vi "Agilent34420-V y HP34401A-R.vi"() -> ()   [LabVIEW 2014]
uses:
  <vilib>/Utility/file.llb/Write To Spreadsheet File (string).vi
  Gonzalo/INTI/Gonzalo/agilent34420_medicion_de_cosa_turbia/Program Files/National Instruments/LabVIEW 2014/instr.lib/Agilent 34401/Agilent 34401.lvlib
panel:
  in  "NPLC Res":sgl(ring)=2.0 format="%_1f" items=["200", "100", "20", "10", "2", "1", ".2", "0.02"]
  out "Res":dbl[](graph)
  in  "GPIB mult 2":refnum<visa-resource-name>="GPIB0::14::INSTR"
  in  "error 2":errorcluster
  in  "t esp medic Res":dbl
  in  "RESOL Res":dbl
  in  "RANGE Res (O)":dbl=0.1
  out "medic Res":dbl[](array[numeric]) format="%#.10e"
  out "Medicion Res":string[](array[string])
  out "Medicion CH1":string[](array[string])
  out "Tmed":string[](array[string])
  out "new file path (Not A Path if cancelled)":path
  out "tiempo transcurrido (s)":dbl
  out "tiempo inicio":timestamp format="%<%H:%M:%S%1u>T"
  in  "t esp medic CH1":dbl
  in  "NPLC CH1":sgl(ring)=2.0 format="%_1f" items=["200", "100", "20", "10", "2", "1", ".2", "0.02"]
  in  "RESOL CH1":dbl
  in  "RANGE CH1 (V)":dbl=0.1
  in  "file path (dialog if empty)":path=path "C:/Users/INTI/Desktop/Gonzalo/INTI/Gonzalo/agilent34420_medicion_de_cosa_turbia/mediciones"
  out "Volt":dbl[](graph)
  out "medic ch 1":dbl[](array[numeric]) format="%#.10e"
  in  "termina medic":bool
  out "Boolean":bool
  in  "empieza medic":bool
  in  "error":errorcluster
  in  "GPIB mult":refnum<visa-resource-name>="GPIB0::13::INSTR"
  # "Notas: el programa mide en forma alternada el canal 1 y 2 del multímetro con los rangos y NPLC seleccionados.\n1- seleccionar GPIB addrs\n2- selccionar RANGE y NPLC de los canales, puede elegirse un file path o dejarlo en blanco (al final se pedirá archivo de datos a grabar).\n3- click en MEDIR para comenzar la medición\n4- click en TERMINAR para finalizarla, se solicita file path en este punto de no haberlo seleccionado previamente."
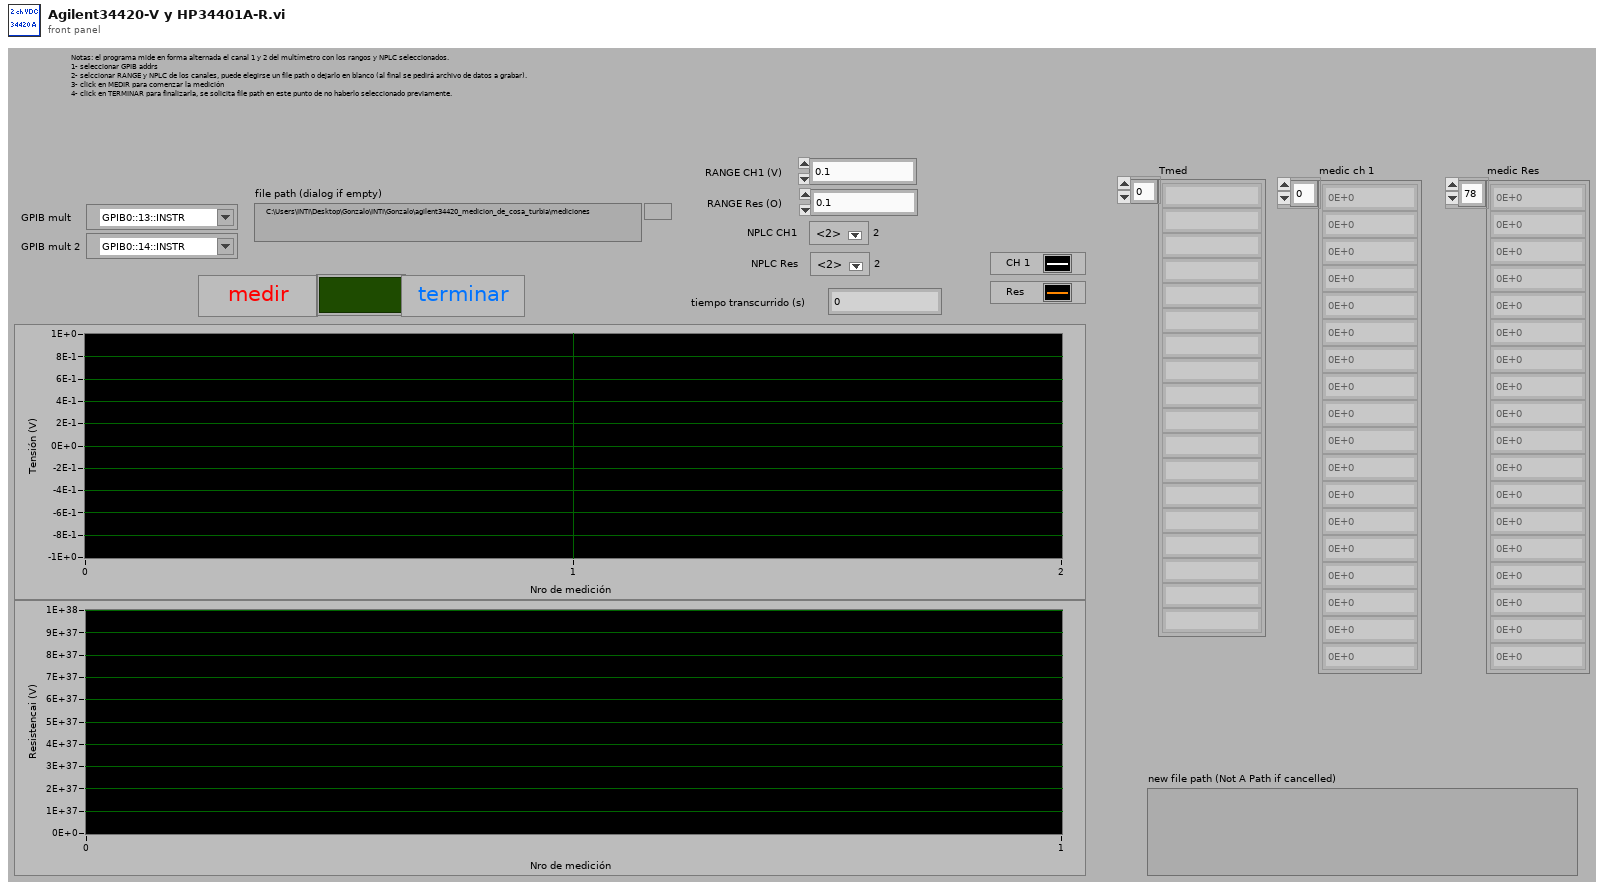
[diagram p1: front panel]
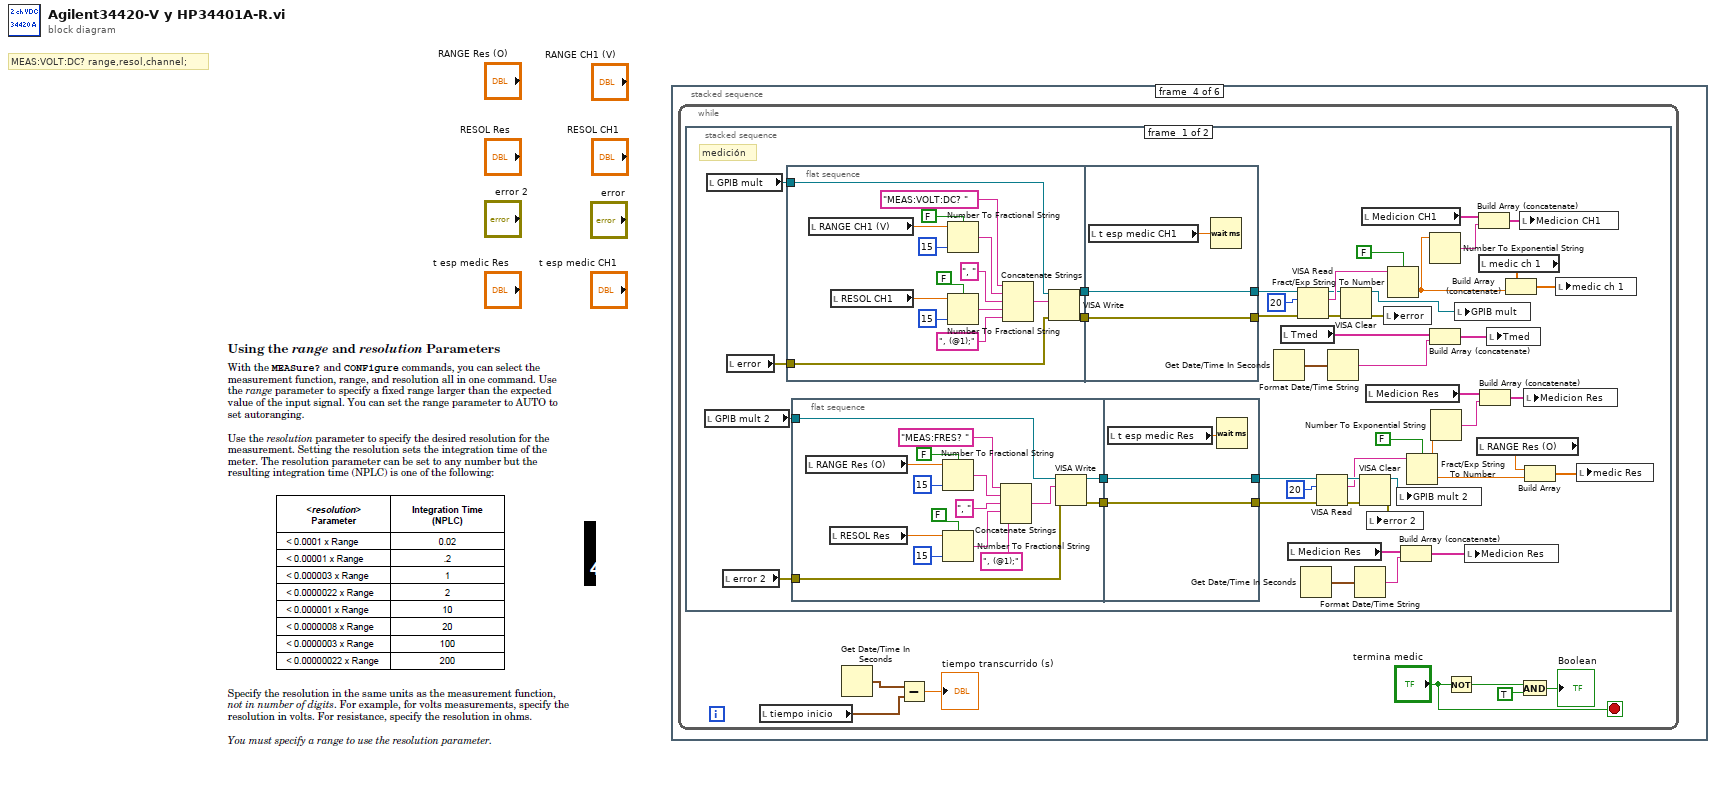
[diagram p0: block diagram]
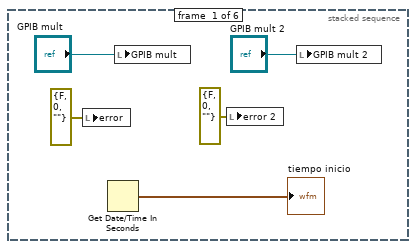
[diagram p2: hidden frame]
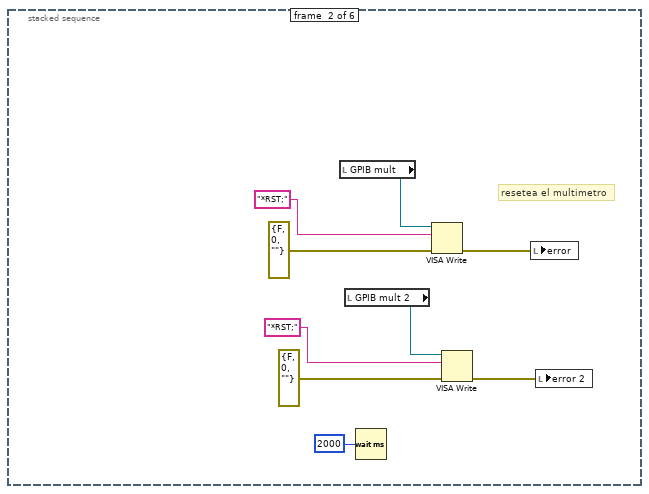
[diagram p3: hidden frame]
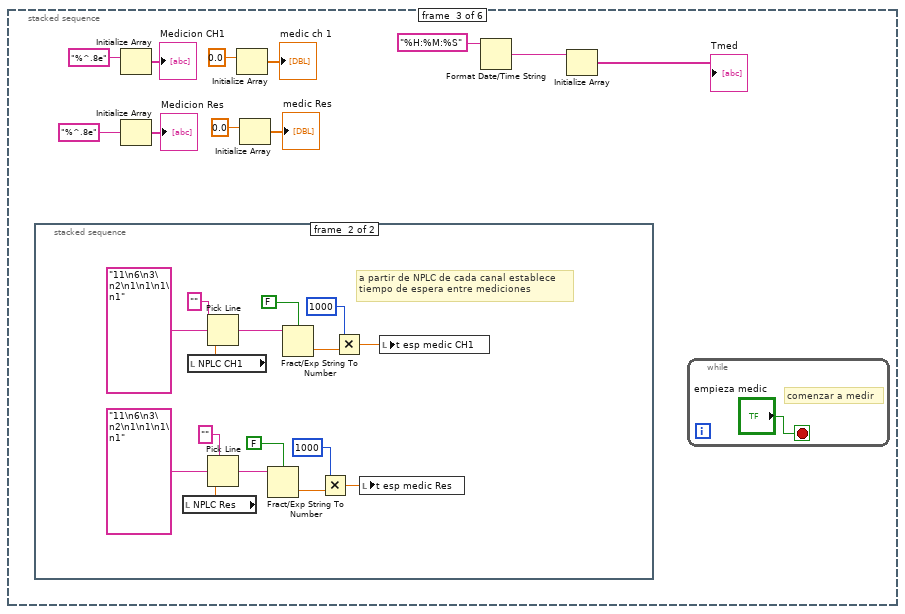
[diagram p4: hidden frame]
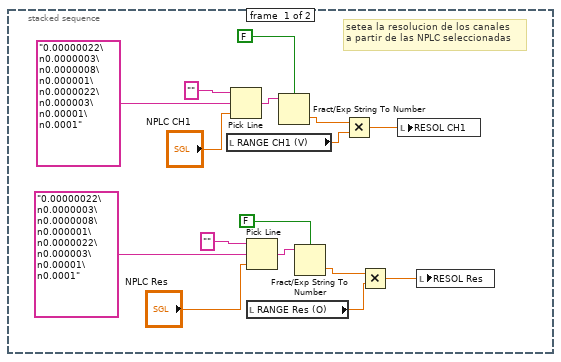
[diagram p5: hidden frame]
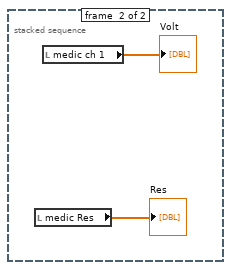
[diagram p6: hidden frame]
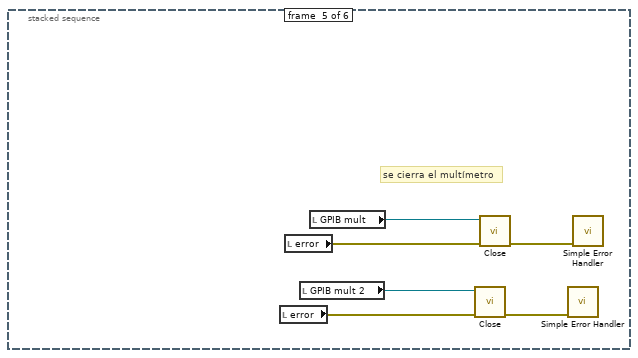
[diagram p7: hidden frame]
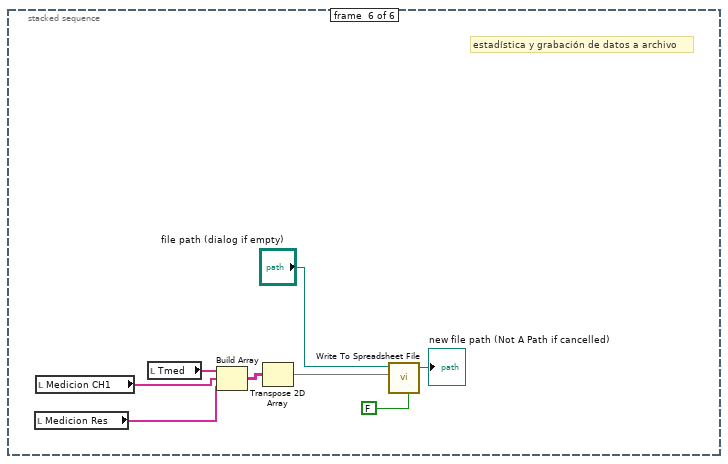
[diagram p8: hidden frame]
diagram:
  # "MEAS:VOLT:DC? range,resol,channel;"
  n1 = stacked-sequence {
    frame #0 {
      n2 = local write "error"(errorcluster {"status"=FALSE, "code"=0, "source"=""} ("error in (no error)")) -> ()
      n3 = Get Date/Time In Seconds() -> (seconds since 1Jan1904=→"tiempo inicio":timestamp)
      n4 = local write "GPIB mult"("GPIB mult") -> ()
      n5 = local write "error 2"(errorcluster {"status"=FALSE, "code"=0, "source"=""} ("error in (no error)")) -> ()
      n6 = local write "GPIB mult 2"("GPIB mult 2") -> ()
    }
    frame #1 {
      # "resetea el multimetro"
      n7 = local read "GPIB mult"() -> (w14:refnum<visa-resource-name>)
      n8 = local read "GPIB mult 2"() -> (w6:refnum<visa-resource-name>)
      n9 = Wait (ms)(milliseconds to wait=u32 2000) -> ()  [unwired: 1 out]
      n10 = VISA Write(VISA resource name=w14, write buffer="*RST;", error in (no error)=errorcluster {"status"=FALSE, "code"=0, "source"=""}) -> (error out=w11:errorcluster)  [unwired: 2 out]
      n11 = VISA Write(VISA resource name=w6, write buffer="*RST;", error in (no error)=errorcluster {"status"=FALSE, "code"=0, "source"=""}) -> (error out=w9:errorcluster)  [unwired: 2 out]
      n12 = local write "error"(w11) -> ()
      n13 = local write "error 2"(w9) -> ()
    }
    frame #2 {
      n14 = stacked-sequence {
        frame #0 {
          # "setea la resolucion de los canales \na partir de las NPLC seleccionadas"
          n15 = local read "RANGE CH1 (V)"() -> (w41:dbl)
          n16 = Pick Line(string ("")="", multi-line string="0.00000022\n0.0000003\n0.0000008\n0.000001\n0.0000022\n0.000003\n0.00001\n0.0001", line index="NPLC CH1") -> (output string=w37:string)
          n17 = Pick Line(string ("")="", multi-line string="0.00000022\n0.0000003\n0.0000008\n0.000001\n0.0000022\n0.000003\n0.00001\n0.0001", line index="NPLC Res") -> (output string=w32:string)
          n18 = local read "RANGE Res (O)"() -> (w27:dbl)
          n19 = Fract/Exp String To Number(use system decimal point (T)=FALSE, string=w37) -> (number=w36:dbl)  [unwired: 2 in, 1 out]
          n20 = Fract/Exp String To Number(use system decimal point (T)=FALSE, string=w32) -> (number=w33:dbl)  [unwired: 2 in, 1 out]
          n21 = Multiply(x=w36, y=w41) -> (x*y=w40:dbl)
          n22 = Multiply(x=w33, y=w27) -> (x*y=w28:dbl)
          n23 = local write "RESOL CH1"(w40) -> ()
          n24 = local write "RESOL Res"(w28) -> ()
        }
        frame #1 {
          # "a partir de NPLC de cada canal establece\ntiempo de espera entre mediciones"
          n25 = local read "NPLC Res"() -> (w42:sgl)
          n26 = local read "NPLC CH1"() -> (w50:sgl)
          n27 = Pick Line(string ("")="", multi-line string="11\n6\n3\n2\n1\n1\n1\n1", line index=w50) -> (output string=w57:string)
          n28 = Pick Line(string ("")="", multi-line string="11\n6\n3\n2\n1\n1\n1\n1", line index=w42) -> (output string=w49:string)
          n29 = Fract/Exp String To Number(use system decimal point (T)=FALSE, string=w49) -> (number=w46:dbl)  [unwired: 2 in, 1 out]
          n30 = Fract/Exp String To Number(use system decimal point (T)=FALSE, string=w57) -> (number=w54:dbl)  [unwired: 2 in, 1 out]
          n31 = Multiply(x=1000, y=w46) -> (x*y=w44:dbl)
          n32 = Multiply(x=1000, y=w54) -> (x*y=w52:dbl)
          n33 = local write "t esp medic Res"(w44) -> ()
          n34 = local write "t esp medic CH1"(w52) -> ()
        }
      }
      n35 = Initialize Array("%^.8e" ("format (%.3f)")) -> (→"Medicion CH1":string[])  [unwired: 1 in]
      n36 = Initialize Array("%^.8e" ("format (%.3f)")) -> (→"Medicion Res":string[])  [unwired: 1 in]
      n37 = Initialize Array(0.0 ("element")) -> (→"medic ch 1":dbl[])  [unwired: 1 in]
      n38 = Initialize Array(0.0 ("element")) -> (→"medic Res":dbl[])  [unwired: 1 in]
      n39 = Format Date/Time String(time format string (%c)="%H:%M:%S") -> (date/time string=w23:string)  [unwired: 2 in]
      n40 = Initialize Array(w23) -> (→"Tmed":string[])  [unwired: 1 in]
      n41 = while {
        stop <- "empieza medic" stop-if-true
        # "comenzar a medir"
      }
    }
    frame #3 {
      n42 = while {
        stop <- "termina medic" stop-if-true
        n43 = stacked-sequence {
          frame #0 {
            # "medición"
            n44 = local read "GPIB mult 2"() -> (w88:refnum<visa-resource-name>)
            n45 = local read "GPIB mult"() -> (w102:refnum<visa-resource-name>)
            n46 = local read "error 2"() -> (w66:errorcluster)
            n47 = local read "error"() -> (w103:errorcluster)
            n48 = flat-sequence {
              tunnel: w103 -> [w146]
              tunnel: w102 -> [w145]
              tunnel: [w144] -> w99
              tunnel: [w143] -> w98
              tunnel: [w148] -> w100
              tunnel: [w149] -> w101
              tunnel: w99 -> [w149]
              tunnel: w98 -> [w148]
              frame #0 {
                n49 = local read "RANGE CH1 (V)"() -> (w141:dbl)
                n50 = local read "RESOL CH1"() -> (w136:dbl)
                n51 = Number To Fractional String(use system decimal point (T)=FALSE, number=w141, precision (6)=i16 15) -> (F-format string=w139:string)  [unwired: 1 in]
                n52 = Number To Fractional String(use system decimal point (T)=FALSE, number=w136, precision (6)=i16 15) -> (F-format string=w135:string)  [unwired: 1 in]
                n53 = Concatenate Strings("MEAS:VOLT:DC? " ("write buffer"), w139, ", " ("string"), w135, ", (@1);" ("string")) -> (w133:string)
                n54 = VISA Write(VISA resource name=w145, write buffer=w133, error in (no error)=w146) -> (VISA resource name out=w144:refnum<visa-resource-name>, error out=w143:errorcluster)  [unwired: 1 out]
              }
              frame #1 {
                n55 = local read "t esp medic CH1"() -> (w147:dbl)
                n56 = Wait (ms)(milliseconds to wait=w147) -> ()  [unwired: 1 out]
              }
            }
            n57 = flat-sequence {
              tunnel: w88 -> [w116]
              tunnel: [w114] -> w87
              tunnel: [w113] -> w86
              tunnel: w66 -> [w112]
              tunnel: w87 -> [w130]
              tunnel: [w130] -> w69
              tunnel: w86 -> [w129]
              tunnel: [w129] -> w68
              frame #0 {
                n58 = local read "RANGE Res (O)"() -> (w119:dbl)
                n59 = local read "RESOL Res"() -> (w124:dbl)
                n60 = Number To Fractional String(use system decimal point (T)=FALSE, number=w119, precision (6)=i16 15) -> (F-format string=w121:string)  [unwired: 1 in]
                n61 = Number To Fractional String(use system decimal point (T)=FALSE, number=w124, precision (6)=i16 15) -> (F-format string=w125:string)  [unwired: 1 in]
                n62 = Concatenate Strings("MEAS:FRES? " ("write buffer"), w121, ", " ("string"), w125, ", (@1);" ("string")) -> (w115:string)
                n63 = VISA Write(VISA resource name=w116, write buffer=w115, error in (no error)=w112) -> (VISA resource name out=w113:refnum<visa-resource-name>, error out=w114:errorcluster)  [unwired: 1 out]
              }
              frame #1 {
                n64 = local read "t esp medic Res"() -> (w128:dbl)
                n65 = Wait (ms)(milliseconds to wait=w128) -> ()  [unwired: 1 out]
              }
            }
            n66 = Get Date/Time In Seconds() -> (seconds since 1Jan1904=w93:timestamp)
            n67 = local read "Tmed"() -> (w95:string[])
            n68 = local read "Medicion Res"() -> (w79:string[])
            n69 = VISA Read(VISA resource name=w101, byte count=u32 20, error in (no error)=w100) -> (VISA resource name out=w109:refnum<visa-resource-name>, read buffer=w111:string, error out=w108:errorcluster)  [unwired: 1 out]
            n70 = Get Date/Time In Seconds() -> (seconds since 1Jan1904=w81:timestamp)
            n71 = VISA Read(VISA resource name=w68, byte count=u32 20, error in (no error)=w69) -> (VISA resource name out=w71:refnum<visa-resource-name>, read buffer=w70:string, error out=w72:errorcluster)  [unwired: 1 out]
            n72 = Format Date/Time String(seconds (now)=w93) -> (date/time string=w94:string)  [unwired: 2 in]
            n73 = VISA Clear(VISA resource name=w109, error in (no error)=w108) -> (VISA resource name out=w106:refnum<visa-resource-name>, error out=w107:errorcluster)
            n74 = Format Date/Time String(seconds (now)=w81) -> (date/time string=w80:string)  [unwired: 2 in]
            n75 = VISA Clear(VISA resource name=w71, error in (no error)=w72) -> (VISA resource name out=w74:refnum<visa-resource-name>, error out=w73:errorcluster)
            n76 = local read "Medicion CH1"() -> (w91:string[])
            n77 = local read "Medicion Res"() -> (w83:string[])
            n78 = local write "error 2"(w73) -> ()
            n79 = local write "error"(w107) -> ()
            n80 = Fract/Exp String To Number(use system decimal point (T)=FALSE, string=w111) -> (number=w92:dbl)  [unwired: 2 in, 1 out]
            n81 = local write "GPIB mult 2"(w74) -> ()
            n82 = Build Array (concatenate)(w79, w80) -> (w78:string[])
            n83 = Fract/Exp String To Number(use system decimal point (T)=FALSE, string=w70) -> (number=w82:dbl)  [unwired: 2 in, 1 out]
            n84 = Number To Exponential String(number=w92) -> (E-format string=w90:string)  [unwired: 3 in]
            n85 = Build Array (concatenate)(w95, w94) -> (w96:string[])
            n86 = Number To Exponential String(number=w82) -> (E-format string=w84:string)  [unwired: 3 in]
            n87 = local write "GPIB mult"(w106) -> ()
            n88 = local write "Medicion Res"(w78) -> ()
            n89 = local read "RANGE Res (O)"() -> (w67:dbl)
            n90 = Build Array (concatenate)(w91, w90) -> (w89:string[])
            n91 = local read "medic ch 1"() -> (w110:dbl[])
            n92 = Build Array (concatenate)(w83, w84) -> (w85:string[])
            n93 = local write "Tmed"(w96) -> ()
            n94 = Build Array (concatenate)(w110, w92) -> (w97:dbl[])
            n95 = local write "Medicion CH1"(w89) -> ()
            n96 = local write "Medicion Res"(w85) -> ()
            n97 = Build Array(w67, w82) -> (w77:dbl[])
            n98 = local write "medic ch 1"(w97) -> ()
            n99 = local write "medic Res"(w77) -> ()
          }
          frame #1 {
            n100 = local read "medic Res"() -> (→"Res":dbl[])
            n101 = local read "medic ch 1"() -> (→"Volt":dbl[])
          }
        }
        n102 = local read "tiempo inicio"() -> (w60:timestamp)
        n103 = Get Date/Time In Seconds() -> (seconds since 1Jan1904=w61:timestamp)
        n104 = Subtract(x=w61, y=w60) -> (x-y=→"tiempo transcurrido (s)":dbl)
        n105 = Not(x="termina medic") -> (.not. x?=w63:bool)
        n106 = And(x=w63, y=TRUE ("Boolean")) -> (x .and. y?=→"Boolean":bool)
      }
    }
    frame #4 {
      # "se cierra el multímetro"
      n107 = local read "error"() -> (w153:errorcluster)
      n108 = local read "error"() -> (w156:errorcluster)
      n109 = local read "GPIB mult 2"() -> (w152:refnum<visa-resource-name>)
      n110 = local read "GPIB mult"() -> (w157:refnum<visa-resource-name>)
      n111 = call "Close.vi"("error in (no error)"=w153, "VISA resource name"=w152) -> ("error out"=w154:errorcluster)  [unwired: 9 in]
      n112 = call "Close.vi"("error in (no error)"=w156, "VISA resource name"=w157) -> ("error out"=w155:errorcluster)  [unwired: 9 in]
      n113 = call <vilib>:"Simple Error Handler.vi"("error in (no error)"=w154) -> ()  [unwired: 4 in, 5 out]
      n114 = call <vilib>:"Simple Error Handler.vi"("error in (no error)"=w155) -> ()  [unwired: 4 in, 5 out]
    }
    frame #5 {
      # "estadística y grabación de datos a archivo"
      n115 = local read "Medicion Res"() -> (w158:string[])
      n116 = local read "Medicion CH1"() -> (w161:string[])
      n117 = local read "Tmed"() -> (w162:string[])
      n118 = Build Array(w162, w161, w158) -> (w160:string[][])
      n119 = Transpose 2D Array(2D array=w160) -> (transposed array=w159:string[][])
      n120 = call-poly <vilib>:"Write To Spreadsheet File.vi"("transpose? (no:F)"=FALSE, "2D data"=w159, "file path (dialog if empty)"="file path (dialog if empty)") -> ("new file path (Not A Path if cancelled)"=→"new file path (Not A Path if cancelled)":path)  [unwired: 5 in]
    }
  }
